vi "RTMain - Top Level.vi"   [LabVIEW 2015]
uses:
  <vilib>/FPGAPlugInAG/myRIO-1900/niLvFpga_Open_myRIO-1900.vi
  <vilib>/rvi/interface/common/dynamic/niFpgaDynamicAddResources.vi
  <vilib>/Utility/error.llb/Error Cluster From Error Code.vi
  <vilib>/rvi/errors/niLvFpgaAdjustHostInterfaceError.vi
  <vilib>/FPGAPlugInAG/Dynamic/niLvFpga_Close_Dynamic.vi
  <vilib>/nisyscfg/Close (System).vi
  <vilib>/rvi/interface/nirviOpenFPGA/nirviOpenFPGA.xnode
  FPGA Bitfiles/WEBUI_FPGATarget_FPGABitfilewithO_5--vQLUfyAg.lvbitx
  FPGA/sample1.vi
  <vilib>/rvi/interface/nirviReadWriteControl/nirviReadWriteControl.xnode
  <vilib>/rvi/interface/nirviCloseFPGA/nirviCloseFPGA.xnode
  <vilib>/nisyscfg/nisyscfg.lvlib
  NiFpgaLv.dll
  <vilib>/rvi/interface/Simulation/niFpgaSimulationCallBeginRW.vi
types:
  T1 = cluster{"Gas Value":dbl, "Knob Value":i16, "DIR":bool, "Stepper ON":bool, "DoorA":bool, "DoorB":bool, "wiper":bool, "Lights 1":bool, "Lights 2":bool, "Turn Signal":i8, "BREAK":bool, "Start Engine":bool, "Undder LIghts":bool}
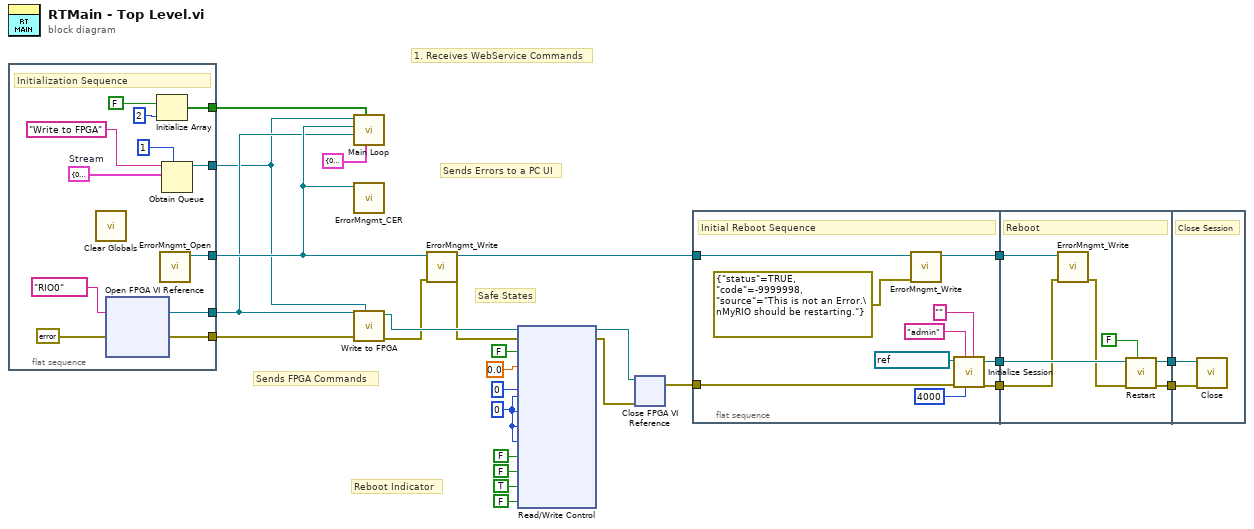
[diagram p0: block diagram]
diagram:
  w21 = u32 0 ("R duty")
  # "Sends FPGA Commands"
  # "Sends Errors to a PC UI"
  # "1. Receives WebService Commands"
  # "Reboot Indicator"
  # "Safe States"
  n1 = flat-sequence {
    tunnel: [w35] -> w15
    tunnel: [w38] -> w5
    tunnel: [w34] -> w4
    tunnel: [w28] -> w2
    tunnel: [w27] -> w1
    frame #0 {
      w31 = T1 {"Gas Value"=0.0, "Knob Value"=0, "DIR"=FALSE, "Stepper ON"=FALSE, "DoorA"=FALSE, "DoorB"=FALSE, "wiper"=FALSE, "Lights 1"=FALSE, "Lights 2"=FALSE, "Turn Signal"=0, "BREAK"=FALSE, "Start Engine"=FALSE, "Undder LIghts"=FALSE}  # Stream
      # "Initialization Sequence"
      n2 = call "Clear Globals.vi"() -> ()  [unwired: 12 in]
      n3 = xnode "Open FPGA VI Reference"("error in"=errorcluster {"status"=FALSE, "code"=0, "source"=""}, "resource name"=tag "RIO0") -> ("FPGA VI Reference Out"=w34:refnum<k20>, "error out"=w35:errorcluster)
      n4 = Initialize Array(FALSE, 2 ("dimension size")) -> (w27:bool[])
      n5 = call "ErrorMngmt_Open.vi"() -> ("Queue out"=w38:refnum<queue>)  [unwired: 10 in, 1 out]
      n6 = Obtain Queue(max queue size (-1, unlimited)=1, name (unnamed)="Write to FPGA", element data type=w31) -> (queue out=w28:refnum<queue>)  [unwired: 2 in, 2 out]
    }
  }
  n7 = call "Main Loop.vi"("Stream"=T1 {"Gas Value"=0.0, "Knob Value"=0, "DIR"=FALSE, "Stepper ON"=FALSE, "DoorA"=FALSE, "DoorB"=FALSE, "wiper"=FALSE, "Lights 1"=FALSE, "Lights 2"=FALSE, "Turn Signal"=0, "BREAK"=FALSE, "Start Engine"=FALSE, "Undder LIghts"=FALSE}, "Array"=w1, "FPGA VI Reference Out"=w4, 10:"Queue in"=w5, 11:"Queue in"=w2) -> ()  [unwired: 7 in]
  n8 = call "ErrorMngmt_CER.vi"("Queue in"=w5) -> ()  [unwired: 11 in]
  n9 = call "Write to FPGA.vi"("Queue in"=w2, "error in (no error)"=w15, "FPGA VI Reference In"=w4) -> ("error out"=w9:errorcluster, "FPGA VI Reference Out"=w10:refnum<k20>)  [unwired: 7 in]
  n10 = call "ErrorMngmt_Write.vi"("error in (no error)"=w9, "Queue in"=w5) -> ("error out"=w8:errorcluster, "Queue out"=w7:refnum<queue>)  [unwired: 8 in]
  n11 = xnode "Read/Write Control"("FPGA VI Reference In"=w10, "error in"=w8, "Stepper ON"=FALSE, "GAS"=sgl 0.0, "Steering"=i16 0, "R duty"=w21, "W duty"=w21, "OL Duty"=w21, "OR Duty"=w21, "LED0"=FALSE, "LED1"=FALSE, "LED2"=TRUE, "LED3"=FALSE) -> ("FPGA VI Reference Out"=w26:refnum<k20>, "error out"=w25:errorcluster)
  n12 = xnode "Close FPGA VI Reference"("FPGA VI Reference In"=w26, "error in"=w25) -> ("error out"=w20:errorcluster)
  n13 = flat-sequence {
    tunnel: w20 -> [w48]
    tunnel: [w46] -> w19
    tunnel: [w45] -> w18
    tunnel: w7 -> [w41]
    tunnel: [w40] -> w6
    tunnel: w19 -> [w55]
    tunnel: w18 -> [w51]
    tunnel: [w54] -> w17
    tunnel: [w53] -> w16
    tunnel: w6 -> [w49]
    tunnel: w17 -> [w57]
    tunnel: w16 -> [w56]
    frame #0 {
      # "Initial Reboot Sequence"
      n14 = call "ErrorMngmt_Write.vi"("error in (no error)"=errorcluster {"status"=TRUE, "code"=-9999998, "source"="This is not an Error.\nMyRIO should be restarting."}, "Queue in"=w41) -> ("Queue out"=w40:refnum<queue>)  [unwired: 8 in, 1 out]
      n15 = call <vilib>:"Initialize Session.vi"("Password"="", "Connect Timeout (4000 ms)"=u32 4000, "User Name"="admin", "error in (no error)"=w48, "Target (localhost)"=refnum<k21> "localhost") -> ("error out"=w45:errorcluster, "Session out"=w46:refnum<k21>)  [unwired: 5 in]
    }
    frame #1 {
      # "Reboot"
      n16 = call "ErrorMngmt_Write.vi"("error in (no error)"=w51, "Queue in"=w49) -> ("error out"=w50:errorcluster)  [unwired: 8 in, 1 out]
      n17 = call <vilib>:"Restart.vi"("Wait Until Complete (T)"=FALSE, "error in (no error)"=w50, "Session in"=w55) -> ("error out"=w54:errorcluster, "Session out"=w53:refnum<k21>)  [unwired: 6 in, 1 out]
    }
    frame #2 {
      # "Close Session"
      n18 = call-poly <vilib>:"Close.vi"("error in (no error)"=w57, "Session in"=w56) -> ()  [unwired: 9 in, 1 out]
    }
  }
